vi "KLF.vi"(0 "System no.":i32=1 min=1 max=4 step=1, 1 "Name":string, 5 "error in":errorcluster) -> (14 "Controller error":bool, 19 "error out":errorcluster)   [LabVIEW 2026]
doc: "Defines a levelling coordinate system (KLF-type) and queries ERR?. A coordinate system defined with this command is intended to eliminate hexapod misalignment. Use KLF in case the hexapod is already in the aligned position. Controller error is TRUE if selected system reports error code not equal to0.\nIf there is already a coordinate system with the same name, KLF will replace it if it is not used. Activating a KLF type coordinate system (KEN.vi) does not cause any motion, and POS?.vi will report new position values. If the hexapod is moving, the command cannot be applied.All pivot point coordinates (SPI.vi) will remain.\"SPI.vi is allowed when a KLF type coordinate system is active. For new or replaced KLF type coordinate systems, the parent coordinate system will be set to \"PI_LEVELLING\".Coordinate system settings are volatile but can be saved as power-on default with WPA.vi using the password \"SKS\".This command requires command level 1 (CCL.vi).\n\nC-887, F-206, M-8X0: Only for GCS syntax version = GCS 2.0 or higher (Check with CSV?.vi. If CSV?.vi is not supported, syntax version is GCS 1.0)."
panel:
  # "Defines a levelling coordinate system (KLF-type) and\nqueries ERR?. A coordinate system defined with this \ncommand is intended to eliminate Hexapod misalignment. \nUse KLF in case the Hexapod is already in the aligned position."
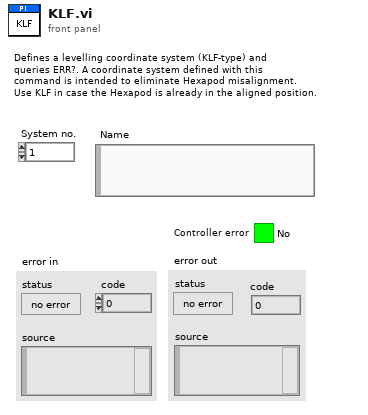
[diagram p1: front panel]
types:
  T1 = enum16{"Disable error check", "Force error check", "Use global settings"}
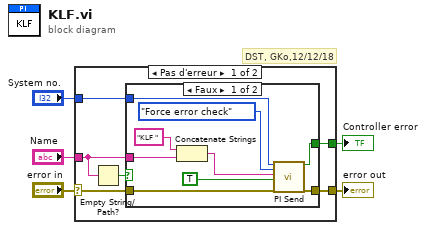
[diagram p0: block diagram]
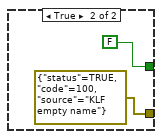
[diagram p2: hidden frame]
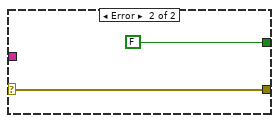
[diagram p3: hidden frame]
diagram:
  # "DST, GKo,12/12/18"
  n1 = case shown="Pas d'erreur" "error in" {
    selector: "error in" -> [w8 w23]
    tunnel: [w11 w23] -> w2
    tunnel: [w10 FALSE ("Controller error")] -> w1
    tunnel: "System no." -> [w9 _]
    tunnel: "Name" -> [w7 _]
    frame No Error {
      n2 = Empty String/Path?(string/path=w7) -> (empty?=w6:bool)
      n3 = case shown="Faux" w6 {
        tunnel: w8 -> [w20 _]
        tunnel: [w15 errorcluster {"status"=TRUE, "code"=100, "source"="KLF empty name"} ("error out")] -> w11
        tunnel: [w14 FALSE ("Controller error")] -> w10
        tunnel: w9 -> [w17 _]
        tunnel: w7 -> [w16 _]
        frame False {
          n4 = Concatenate Strings("KLF ", w16) -> (w18:string)
          n5 = call "PI Send.vi"("System no."=w17, "Error check settings"=T1."Force error check", "String to send"=w18, "Attach termination char.?"=TRUE ("Attach Linefeed?"), "error in"=w20) -> ("Controller error"=w14:bool, "error out"=w15:errorcluster)  [unwired: 1 in, 12 out]
        }
        frame True {
        }
      }
    }
    frame Error {
    }
  }
  "error out" <- w2
  "Controller error" <- w1
